vi "GetHelp.vi"(11 "LUnitCLI in":refnum<class "LUnitCLI.lvclass">) -> (2 "Help":string, 3 "LUnitCLI out":refnum<class "LUnitCLI.lvclass">)   [LabVIEW 2020, in "LUnitCLI.lvclass"]
uses:
  LUnitCLI.lvclass
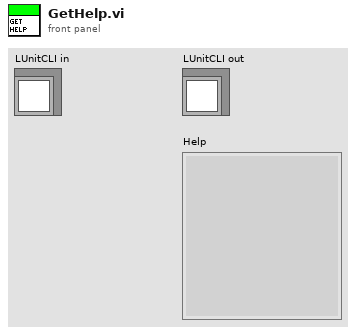
[diagram p1: front panel]
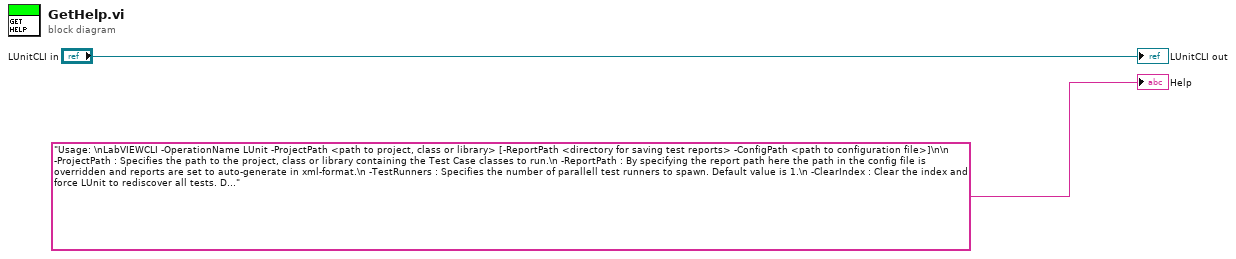
[diagram p0: block diagram]
diagram:
  "LUnitCLI out" <- "LUnitCLI in"
  "Help" <- "Usage: \nLabVIEWCLI -OperationName LUnit -ProjectPath <path to project, class or library> [-ReportPath <directory for saving test reports> -ConfigPath <path to configuration file>]\n\n -ProjectPath : Specifies the path to the project, class or library containing the Test Case classes to run.\n -ReportPath : By specifying the report path here the path in the config file is overridden and reports are set to auto-generate in xml-format.\n -TestRunners : Specifies the number of parallell test runners to spawn. Default value is 1.\n -ClearIndex : Clear the index and force LUnit to rediscover all tests. Default is True."
